vi "S2C_PCIe1762H_Proc_ResetAll.vi"(8 "Error In":errorcluster) -> (0 "Error Out":errorcluster)   [LabVIEW 2024]
uses:
  S2C_PCIe1762H_Proc_Globals.vi
  <userlib>/DAQNavi Polymorphic VI/create/DAQNavi Create Channel(DO-Digital Output).vi
  <userlib>/DAQNavi Polymorphic VI/write/DAQNavi Write (Digtial 1D U8 NChan 1Samp).vi
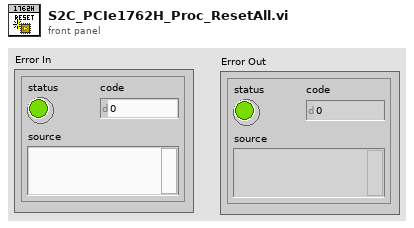
[diagram p1: front panel]
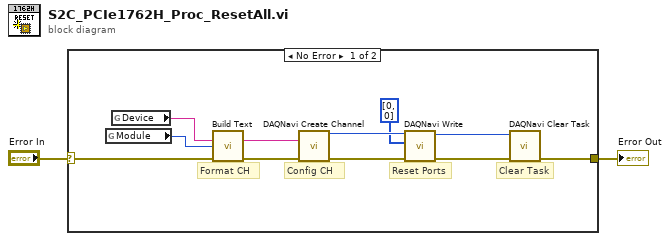
[diagram p0: block diagram]
diagram:
  n1 = case shown="No Error" "Error In" {
    selector: "Error In" -> [w9 w14]
    tunnel: [w3 w14] -> w1
    frame No Error {
      # "Reset Ports"
      # "Clear Task"
      # "Format CH"
      # "Config CH"
      n2 = global read "S2C_PCIe1762H_Proc_Globals.vi" "Module"() -> (w12:i32)
      n3 = global read "S2C_PCIe1762H_Proc_Globals.vi" "Device"() -> (w13:string)
      n4 = call "Build Text"("Device"=w13, "Module"=w12, "error in (no error)"=w9) -> ("Result"=w11:string, "error out"=w10:errorcluster)  [unwired: 11 in]
      n5 = call-poly <userlib>:"DAQNavi Create Channel.vi"("physical channels"=w11, "error in (no error)"=w10) -> ("task out"=w7:i32, "error out"=w8:errorcluster)  [unwired: 3 in, 9 out]
      n6 = call-poly <userlib>:"DAQNavi Write.vi"("error in (no error)"=w8, "data"=u8[] [0, 0], "task in"=w7) -> ("error out"=w5:errorcluster, "task out"=w4:i32)  [unwired: 6 in, 1 out]
      n7 = call <userlib>:"DAQNavi Clear Task.vi"("error in (no error)"=w5, "task in"=w4) -> ("error out"=w3:errorcluster)  [unwired: 1 out]
    }
    frame Error {
    }
  }
  "Error Out" <- w1
